vi "Decode Frame ID.vi"(11 "Frame ID in":u32) -> (1 "ISO FD Type":T1=enum."CAN 2.0", 2 "Extended ID":bool, 3 "Frame ID out":u32)   [LabVIEW 2021, in "CAN_Logic.lvclass"]
uses:
  CAN_Logic.lvclass
  typedef/ISO FD Frame Type.ctl
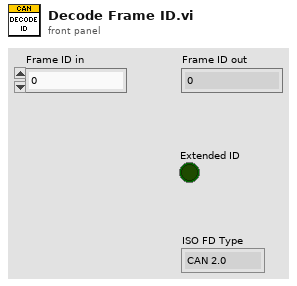
[diagram p1: front panel]
types:
  T1 = typedef "CAN_Logic.lvclass/ISO FD Frame Type.ctl" = enum16{"Not Specified", "CAN 2.0", "FD", "FD+BRS"}
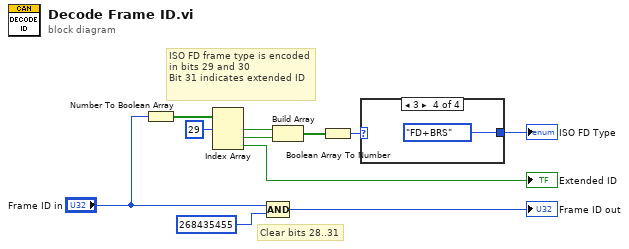
[diagram p0: block diagram]
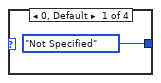
[diagram p2: hidden frame]
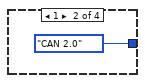
[diagram p3: hidden frame]
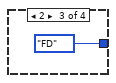
[diagram p4: hidden frame]
diagram:
  # "Clear bits 28..31"
  # "ISO FD frame type is encoded in bits 29 and 30\nBit 31 indicates extended ID"
  n1 = Number To Boolean Array(number="Frame ID in") -> (Boolean array=w11:bool[])
  n2 = Index Array(array=w11, index #1=29 ("index")) -> (element #1=w5:bool, element #2=w4:bool, element #3=→"Extended ID":bool)  [unwired: 2 in]
  n3 = Compound Arithmetic op=AND("Frame ID in", u32 268435455 ("value")) -> (→"Frame ID out":u32)
  n4 = Build Array(w5, w4) -> (w3:bool[])
  n5 = Boolean Array To Number(Boolean array=w3) -> (number=w2:u8)
  n6 = case shown="3" w2 {
    tunnel: [ISO_FD_Frame_Type."Not Specified" ("ISO FD Type 2") ISO_FD_Frame_Type."CAN 2.0" ("ISO FD Type 2") ISO_FD_Frame_Type."FD" ("ISO FD Type 2") ISO_FD_Frame_Type."FD+BRS" ("ISO FD Type 2")] -> w1
    frame 0, Default {
    }
    frame 1 {
    }
    frame 2 {
    }
    frame 3 {
    }
  }
  "ISO FD Type" <- w1
